vi "Cleaning Service.vi"() -> ()   [LabVIEW 2023]
panel:
  out "Status 6":bool
  out "Status 5":bool
  out "Status 4":bool
  out "Status 3":bool
  out "Status 2":bool
  out "Status 1":bool
  in  "Hotel":string
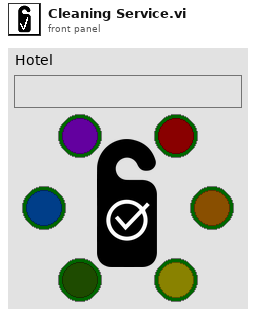
[diagram p1: front panel]
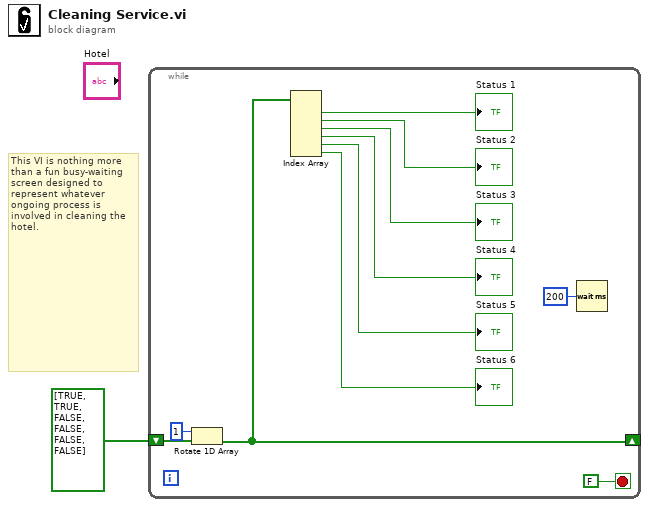
[diagram p0: block diagram]
diagram:
  # "This VI is nothing more than a fun busy-waiting screen designed to represent whatever ongoing process is involved in cleaning the hotel."
  n1 = while {
    shift-right: [w9] -> _
    shift-left: bool[] [TRUE, TRUE, FALSE, FALSE, FALSE, FALSE] -> [w11]
    stop <- FALSE stop-if-true
    n2 = Rotate 1D Array(1:w11, 2:1 ("n")) -> (0:w9:bool[])
    n3 = Index Array(array=w9) -> (element #1=→"Status 1":bool, element #2=→"Status 2":bool, element #3=→"Status 3":bool, element #4=→"Status 4":bool, element #5=→"Status 5":bool, element #6=→"Status 6":bool)  [unwired: 6 in]
    n4 = Wait (ms)(milliseconds to wait=u32 200) -> ()  [unwired: 1 out]
  }
